vi "Set Mode.vi"(8 "error in (no error)":errorcluster, 10 "TCP Mode":T1, 11 "TCP Client in":refnum<class "TCP Client.lvclass">) -> (0 "error out":errorcluster, 3 "TCP Client out":refnum<class "TCP Client.lvclass">)   [LabVIEW 2020, in "Stream-TCP.lvlib" / "TCP Client.lvclass"]
uses:
  TCP Client.lvclass
  TCP Mode.ctl
  TCP Client.lvclass/TCP Client.ctl
  Stream-TCP.lvlib
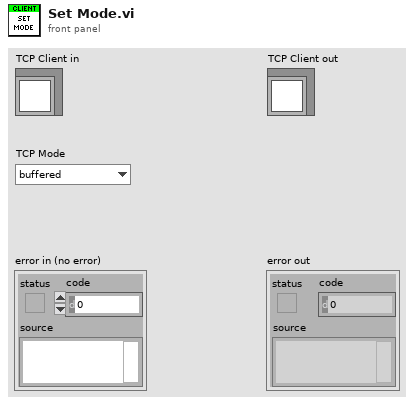
[diagram p1: front panel]
types:
  T1 = typedef "Stream-TCP.lvlib/TCP Mode.ctl" = enum16{"buffered", "raw"}
  T2 = typedef "Stream-TCP.lvlib/TCP Client.lvclass/Ref Data.ctl" = cluster{"TCP Connection":refnum<k5>, "TCP Stream":refnum<class "TCP Stream.lvclass">, "State":T3, "Connection Loop":refnum<vi>, "TCP Mode":T1, "Timeout ms":i32}
  T3 = typedef "Stream-TCP.lvlib/TCP Client.lvclass/Connection State.ctl" = enum16{"Closed", "Idle", "Connecting", "Connected", "Shutdown"}
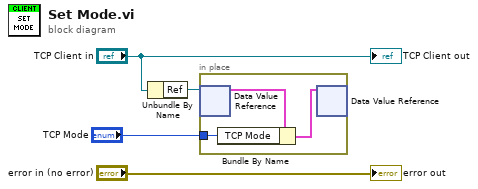
[diagram p0: block diagram]
diagram:
  n1 = Unbundle By Name("TCP Client in") -> ("Ref"=w3:refnum<data-value>)
  n2 = in-place {
    in-place-border: "TCP Mode" -> [w5]
    n3 = in-place-dvr #1(w3) -> (w7:T2)  [unwired: 1 out]
    n4 = Bundle By Name(cluster=w7, "TCP Mode"=w5) -> (w6:T2)
    n5 = in-place-dvr #1(w6) -> ()  [unwired: 2 out]
  }
  "error out" <- "error in (no error)"
  "TCP Client out" <- "TCP Client in"
